vi "Write Binary Recovery File.vi"(8 "error in (no error)":errorcluster, 10 "Data In":dbl[](array[numeric]), 11 "Path":path) -> (0 "error out":errorcluster)   [LabVIEW 2020]
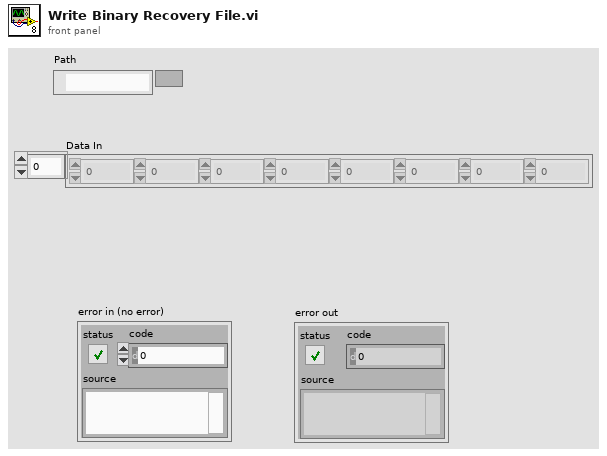
[diagram p1: front panel]
types:
  T1 = enum16{"open", "replace", "create", "open or create", "replace or create", "replace or create with confirmation"}
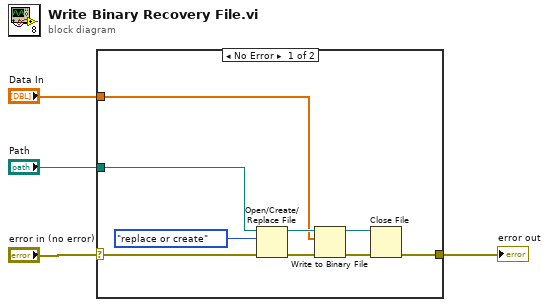
[diagram p0: block diagram]
diagram:
  n1 = case shown="No Error" "error in (no error)" {
    selector: "error in (no error)" -> [w12 w14]
    tunnel: "Path" -> [w13 _]
    tunnel: [w11 w14] -> w2
    tunnel: "Data In" -> [w6 _]
    frame No Error {
      n2 = Open/Create/Replace File(file path (use dialog)=w13, error in=w12, operation (0:open)=T1."replace or create") -> (refnum out=w10:refnum<file>, error out=w9:errorcluster)  [unwired: 3 in, 1 out]
      n3 = Write to Binary File(file (use dialog)=w10, data=w6, error in=w9) -> (refnum out=w8:refnum<file>, error out=w7:errorcluster)  [unwired: 3 in, 1 out]
      n4 = Close File(refnum=w8, error in=w7) -> (error out=w11:errorcluster)  [unwired: 1 out]
    }
    frame Error {
    }
  }
  "error out" <- w2
